vi "_AttributeDataType.vi"(2 "attribute name":string, 3 "device name":string) -> (0 "data type value":u16=36, 1 "data type enum":T1=enum."UNKNOWN_DATA_TYPE")   [LabVIEW 2014, in "tango.lvlib"]
uses:
  tango.lvlib
  Common VIs/Typedefs/_AttributeDataType_t.ctl
  tango_binding.so
panel:
  out "error_stack":string[](array[string])
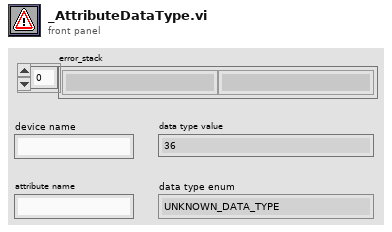
[diagram p1: front panel]
types:
  T1 = typedef "tango.lvlib/_AttributeDataType_t.ctl" = enum16{"STATE_SCA", "STATE_SPE", "STATE_IMG", "STRING_SCA", "STRING_SPE", "STRING_IMG", "BOOL_SCA", "BOOL_SPE", "BOOL_IMG", "UCHAR_SCA", "UCHAR_SPE", "UCHAR_IMG", "SHORT_SCA", "SHORT_SPE", "SHORT_IMG", "USHORT_SCA", "USHORT_SPE", "USHORT_IMG", "LONG_SCA", "LONG_SPE", "LONG_IMG", "ULONG_SCA", "ULONG_SPE", "ULONG_IMG", "LONG64_SCA", "LONG64_SPE", "LONG64_IMG", "ULONG64_SCA", "ULONG64_SPE", "ULONG64_IMG", "FLOAT_SCA", "FLOAT_SPE", "FLOAT_IMG", "DOUBLE_SCA", "DOUBLE_SPE", "DOUBLE_IMG", "UNKNOWN_DATA_TYPE"}
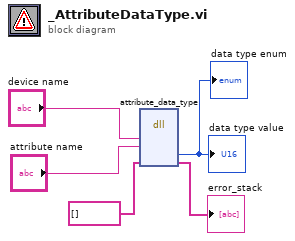
[diagram p0: block diagram]
diagram:
  n1 = dll-call lib="tango_binding.*" fn="attribute_data_type"("device_name"="device name", "attribute_name"="attribute name", "error_stack"=string[] [] ("error stack")) -> ("data_type"=→"data type value" →"data type enum":u32, "error_stack"=→"error_stack":string[])  [unwired: 7 in, 2 out]
